vi "PSU.vi"(1 "Up":u16 max=1000, 2 "Ie":u8=1 min=1 max=20) -> (0 "data string":string)   [LabVIEW 2012]
panel:
  out "*(type *) &x":string
  out "4 bajt":bool[](array[boolean])
  out "3 bajt":bool[](array[boolean])
  out "2 bajt":bool[](array[boolean])
  out "1 bajt":bool[](array[boolean])
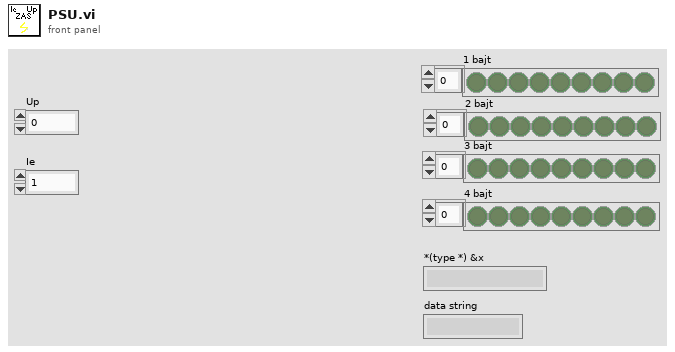
[diagram p1: front panel]
types:
  T1 = enum16{"big-endian, network order", "native, host order", "little-endian"}
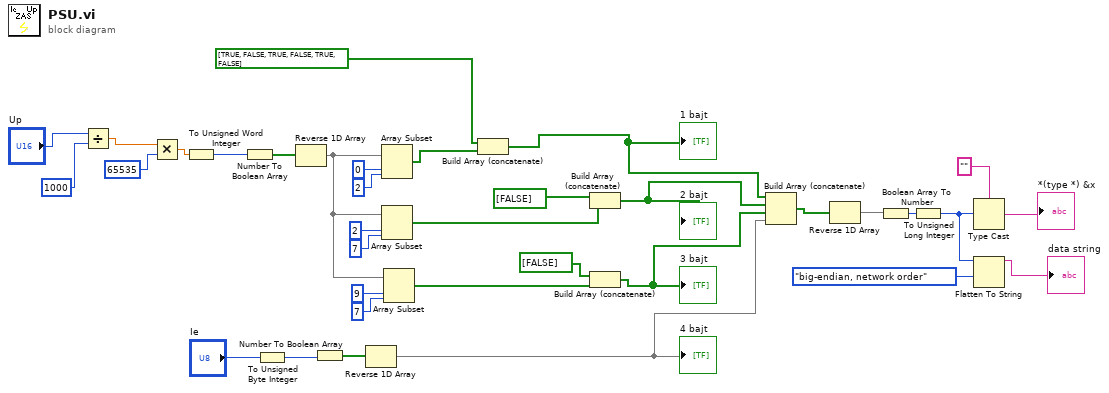
[diagram p0: block diagram]
diagram:
  n1 = Divide(x="Up", y=u16 1000) -> (x/y=w3:dbl)
  n2 = Multiply(x=w3, y=u16 65535) -> (x*y=w2:dbl)
  n3 = To Unsigned Word Integer(number=w2) -> (unsigned 16bit integer=w12:u16)
  n4 = Number To Boolean Array(number=w12) -> (Boolean array=w35:bool[])
  n5 = To Unsigned Byte Integer(number="Ie") -> (unsigned 8bit integer=w9:u8)
  n6 = Reverse 1D Array(array=w35) -> (reversed array=w1:bool[])
  n7 = Number To Boolean Array(number=w9) -> (Boolean array=w34:bool[])
  n8 = Reverse 1D Array(array=w34) -> (reversed array=w20:bool[])
  "4 bajt" <- w20
  n9 = Array Subset(array=w1, index=0, length=2) -> (w31:bool[])
  n10 = Array Subset(array=w1, index=2, length=7) -> (w28:bool[])
  n11 = Array Subset(array=w1, index=9, length=7) -> (w23:bool[])
  n12 = Build Array (concatenate)(bool[] [TRUE, FALSE, TRUE, FALSE, TRUE, FALSE] ("array"), w31) -> (w10:bool[])
  "1 bajt" <- w10
  n13 = Build Array (concatenate)(bool[] [FALSE] ("array"), w28) -> (w22:bool[])
  "2 bajt" <- w22
  n14 = Build Array (concatenate)(bool[] [FALSE] ("array"), w23) -> (w21:bool[])
  "3 bajt" <- w21
  n15 = Build Array (concatenate)(w10, w22, w21, w20) -> (w19:bool[])
  n16 = Reverse 1D Array(array=w19) -> (reversed array=w18:bool[])
  n17 = Boolean Array To Number(Boolean array=w18) -> (number=w6:u32)
  n18 = To Unsigned Long Integer(number=w6) -> (unsigned 32bit integer=w7:u32)
  n19 = Type Cast(type="", x=w7) -> (*(type *) &x=→"*(type *) &x":string)
  n20 = Flatten To String(anything=w7, byte order (0:big-endian, network order)=T1."big-endian, network order") -> (data string=→"data string":string)  [unwired: 2 in, 2 out]
